vi "Check Tool Type.vi"(11 "Tool Config Cluster":T1={"Tool Type"=0, "Tool SN"=0, "Tool Block"={"Encoder Size"=0, "Encoder Scale"=0, "Encoder Offset"=0, "MaxEncoder"=0, "MinEncoder"=0, "Start Delay"=0.0, "Tool Face Ref"=0.0}, "Motor Block"={"MinMotor Speed"=0, "MaxMotor Speed"=0, "Homing Speed"=90, "Jog Speed"=90, "Inspect Speed"=90, "VBlk Speed"=90, "CleaningPos"=0, "Safe Zone"=0, "Has Motor"=FALSE, "Use Home Index"=FALSE}, "Verification Block"={"Angle"=90.0, "FlankLength1"=0.0, "FlankLength2"=0.0, "Location"=0.0, "Serial Number"=0}, "Probe Block"={"nProbes"=0, "Probe Param Array"=[]}} {"Probe Block"."Probe Param Array"."Sensor Block"."SensorCfgParams Array"."CalibrCoefArray" format="%#.12g"}) -> (2 "Success":bool, 3 "Tool Type":u16)   [LabVIEW 2015, in "Tool Module.lvlib"]
uses:
  Tool Module.lvlib
  Tool Config/_Configuration Cluster_v3--typedef.ctl
  Tool Config/_Tool Block Cluster_v3--typedef.ctl
  Tool Config/_Motor Block Cluster_v2--typedef.ctl
  Tool Config/_Verification Blk Cluster--typedef.ctl
  Tool Config/_ProbeConfigParams Cluster--typedef.ctl
  Tool Config/_Sensor Block Cluster--typedef.ctl
  Tool Config/_SensorConfigParams Cluster--typedef.ctl
  Tool Config/Tool Cfg.lvlib
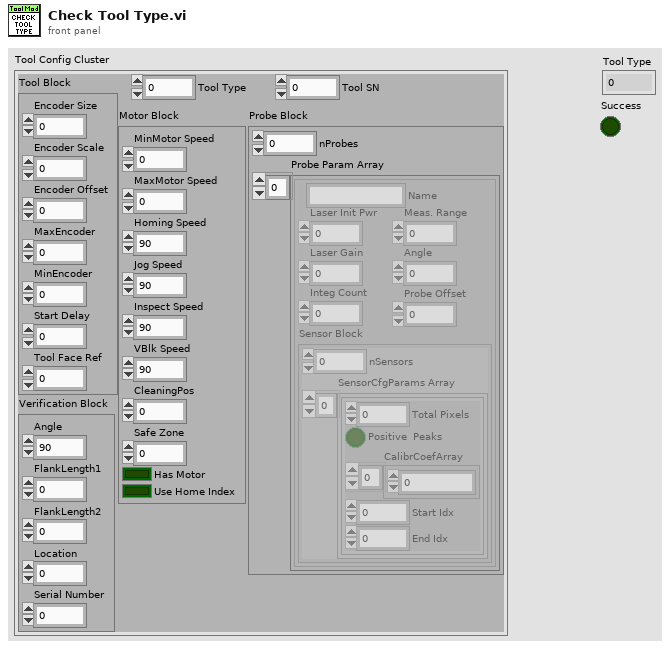
[diagram p1: front panel]
types:
  T1 = typedef "Tool Cfg.lvlib/_Configuration Cluster_v3--typedef.ctl" = cluster{"Tool Type":u16, "Tool SN":u16, "Tool Block":T2, "Motor Block":T3, "Verification Block":T4, "Probe Block":cluster{"nProbes":u16, "Probe Param Array":T5[]}}
  T2 = typedef "Tool Cfg.lvlib/_Tool Block Cluster_v3--typedef.ctl" = cluster{"Encoder Size":u16, "Encoder Scale":u32, "Encoder Offset":i32, "MaxEncoder":i32, "MinEncoder":i32, "Start Delay":sgl, "Tool Face Ref":sgl}
  T3 = typedef "Tool Cfg.lvlib/_Motor Block Cluster_v2--typedef.ctl" = cluster{"MinMotor Speed":u16, "MaxMotor Speed":u16, "Homing Speed":u16, "Jog Speed":u16, "Inspect Speed":u16, "VBlk Speed":u16, "CleaningPos":i32, "Safe Zone":i32, "Has Motor":bool, "Use Home Index":bool}
  T4 = typedef "Tool Cfg.lvlib/_Verification Blk Cluster--typedef.ctl" = cluster{"Angle":sgl, "FlankLength1":sgl, "FlankLength2":sgl, "Location":sgl, "Serial Number":u16}
  T5 = typedef "Tool Cfg.lvlib/_ProbeConfigParams Cluster--typedef.ctl" = cluster{"Name":string, "Laser Init Pwr":u16, "Laser Gain":u8, "Integ Count":u16, "Meas. Range":sgl, "Angle":sgl, "Probe Offset":sgl, "Sensor Block":T6}
  T6 = typedef "Tool Cfg.lvlib/_Sensor Block Cluster--typedef.ctl" = cluster{"nSensors":u16, "SensorCfgParams Array":T7[]}
  T7 = typedef "Tool Cfg.lvlib/_SensorConfigParams Cluster--typedef.ctl" = cluster{"Total Pixels":u16, "Positive  Peaks":bool, "CalibrCoefArray":dbl[], "Start Idx":u16, "End Idx":u16}
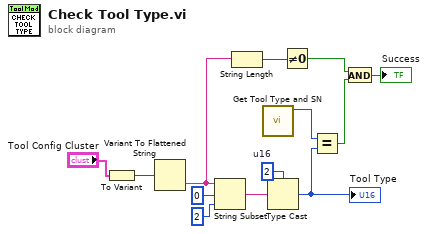
[diagram p0: block diagram]
diagram:
  w9 = u16 2  # u16
  n1 = To Variant(anything="Tool Config Cluster") -> (Variant=w5:variant)
  n2 = Variant To Flattened String(Variant=w5) -> (data string=w13:string)  [unwired: 1 out]
  n3 = String Subset(string=w13, offset (0)=0, length (rest)=2 ("length (rest)")) -> (substring=w6:string)
  n4 = String Length(string=w13) -> (length=w12:i32)
  n5 = call "Get Tool Type and SN.vi"() -> ("Tool Type"=w1:u16)  [unwired: 10 in, 1 out]
  n6 = Type Cast(type=w9, x=w6) -> (*(type *) &x=w3:u16)
  "Tool Type" <- w3
  n7 = Not Equal To 0?(x=w12) -> (x != 0?=w11:bool)
  n8 = Equal?(x=w1, y=w3) -> (x = y?=w2:bool)
  n9 = And(x=w11, y=w2) -> (x .and. y?=→"Success":bool)
